vi "setRampTime.vi"(8 "error in (no error)":errorcluster, 10 "rampTime":dbl, 11 "SingleToneRamp.lvclass in":refnum<class "SingleToneRamp.lvclass">) -> (0 "error out":errorcluster, 3 "SingleToneRamp.lvclass out":refnum<class "SingleToneRamp.lvclass">)   [LabVIEW 2011, in "Tools.lvlib" / "Scripting.lvlib" / "SingleToneRamp.lvclass"]
uses:
  SingleToneRamp.lvclass
  SingleToneRamp.lvclass/SingleToneRamp.ctl
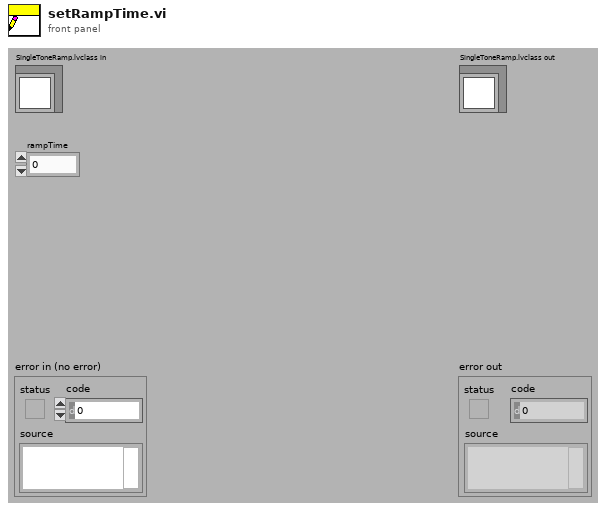
[diagram p1: front panel]
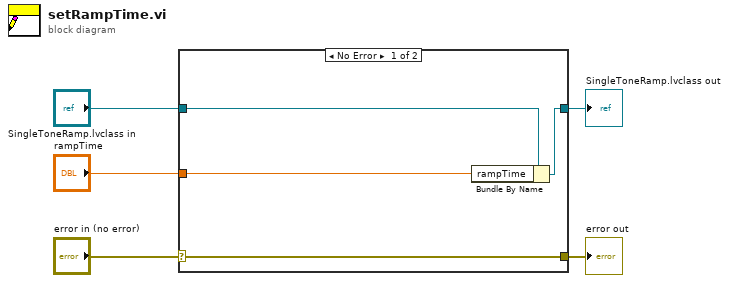
[diagram p0: block diagram]
diagram:
  n1 = case shown="No Error" "error in (no error)" {
    selector: "error in (no error)" -> [w9 w10]
    tunnel: [w9 w10] -> w4
    tunnel: [w7 w11] -> w2
    tunnel: "SingleToneRamp.lvclass in" -> [w8 w11]
    tunnel: "rampTime" -> [w6 _]
    frame No Error {
      n2 = Bundle By Name(cluster=w8, "rampTime"=w6) -> (w7:refnum<class "SingleToneRamp.lvclass">)
    }
    frame Error {
    }
  }
  "error out" <- w4
  "SingleToneRamp.lvclass out" <- w2
